vi "V1_controls.vi"() -> ()   [LabVIEW 2020]
uses:
  C:/Users/359167/Documents/LabVIEW_ws/Thorlabs.MotionControl.FTD2xx_Net.dll
  Thorlabs.MotionControl.FTD2xx_Net.dll
  <vilib>/DAQmx/read.llb/DAQmx Read (Analog 1D Wfm NChan NSamp).vi
panel:
  in  "Run":bool
  in  "End":bool
  out "Device ID":string[](array[string])
  out "Serial Number":string[](array[string])
  out "Voltage":dbl[][](array[numeric])
  out "Array":string[][](array[string])
  out "mount labels":string[](array[string])
  out "DAQ channels":string[](array[string])
  out "# of channels":i32
  out "voltage vs. time":waveform(dbl)[](graph) caption="data"
  out "# of mounts":i32
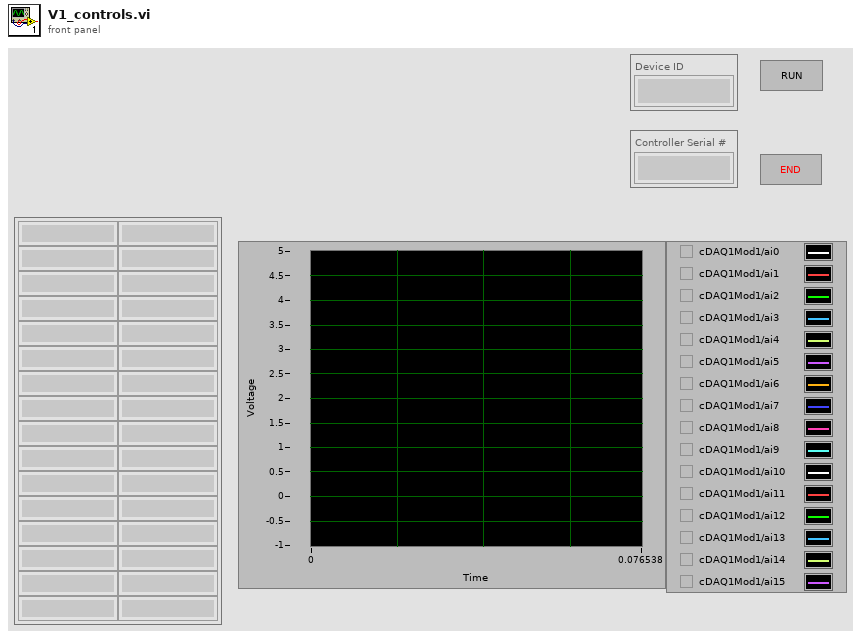
[diagram p1: front panel]
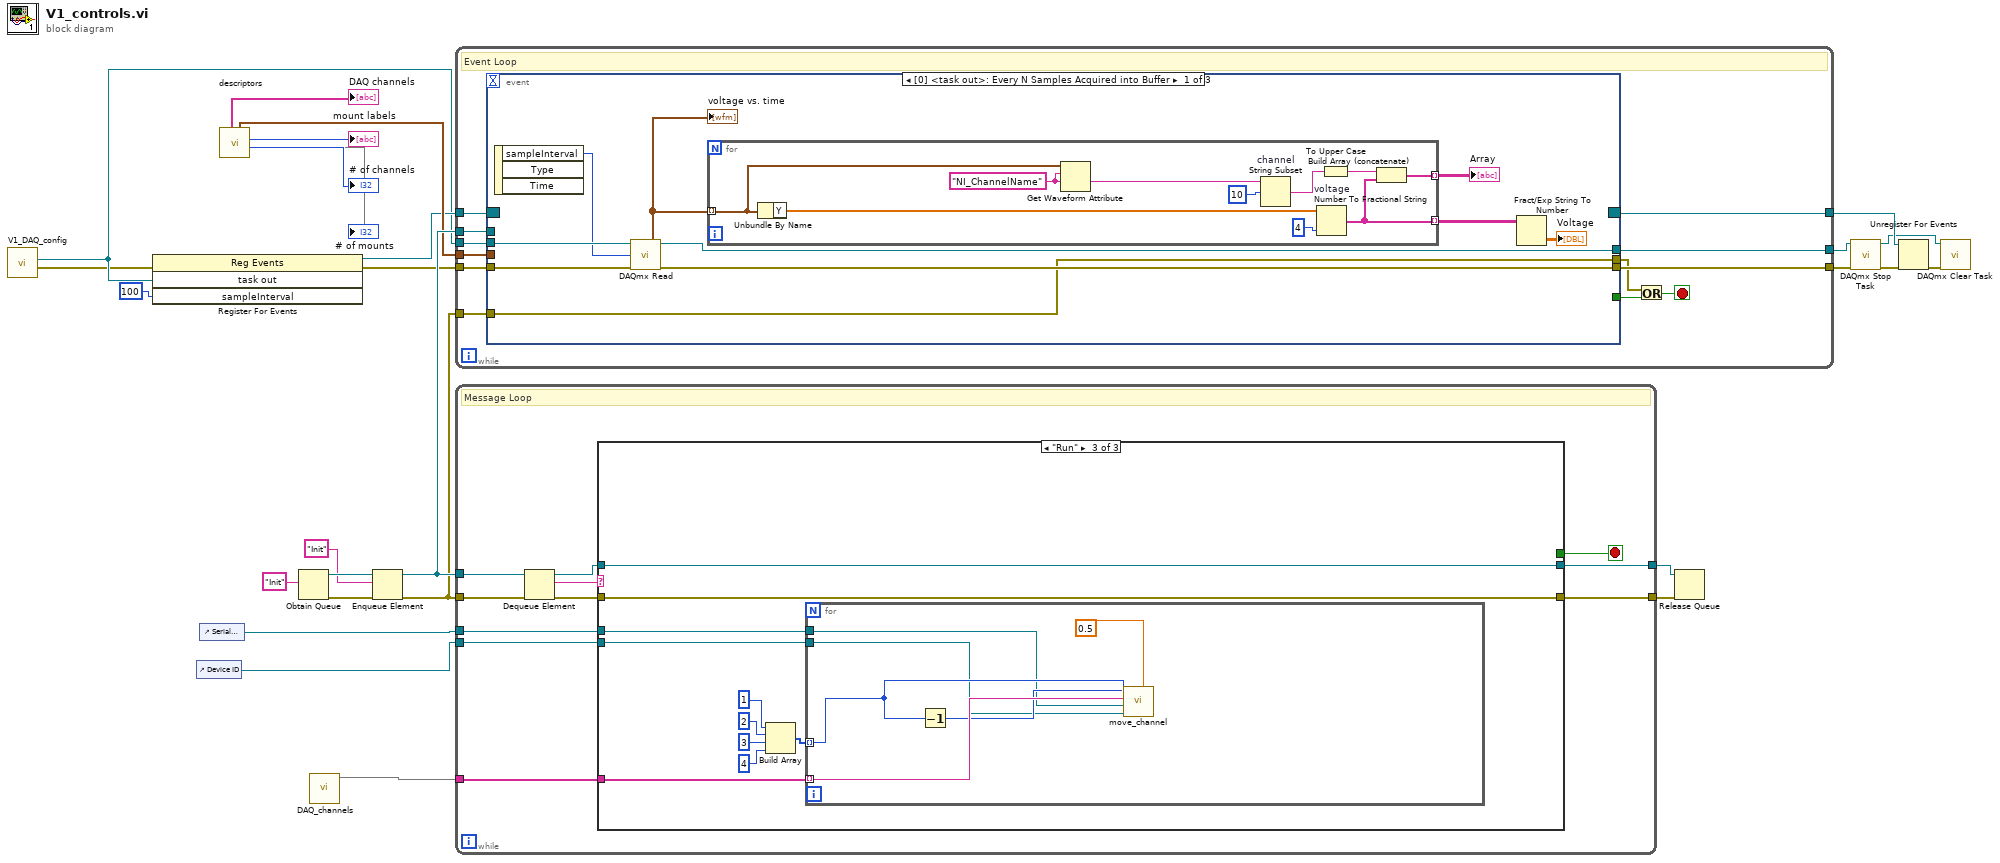
[diagram p0: block diagram]
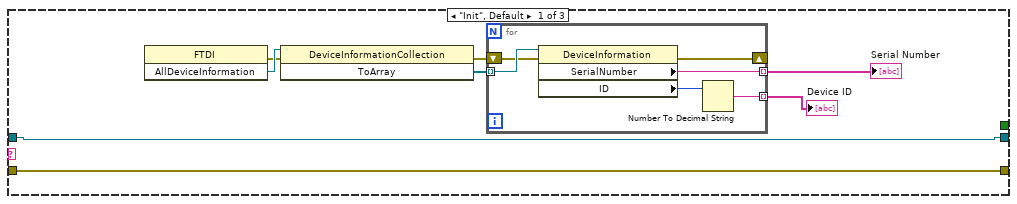
[diagram p2: hidden frame]
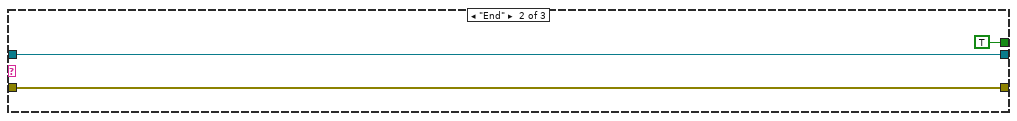
[diagram p3: hidden frame]
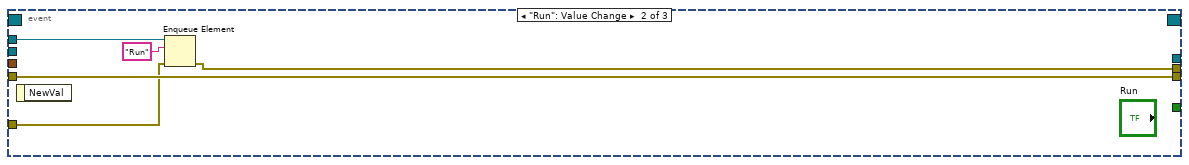
[diagram p4: hidden frame]
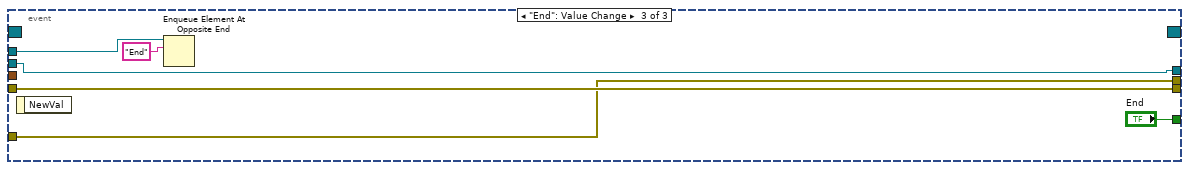
[diagram p5: hidden frame]
diagram:
  n1 = call "V1_DAQ_config.vi"() -> ("error out"=w7:errorcluster, "task out"=w12:refnum<k21>)  [unwired: 10 in]
  n2 = register-events(error in=w7, w12, u32 100 ("sampleInterval")) -> (reference out=w13:refnum<event-registration>, error out=w6:errorcluster)  [unwired: 1 in]
  n3 = control-ref of="Device ID"() -> (w1:refnum<vi>)
  n4 = control-ref of="Serial Number"() -> (w2:refnum<vi>)
  n5 = call "descriptors.vi"() -> ("# of channels"=→"# of channels":i32, "# of controllers"=→"mount labels":i32, 4:→"# of mounts", "channel pairs"=w21:cluster{i32, i32}[], "DAQ channels"=→"DAQ channels":string[])  [unwired: 6 in, 1 out]
  n6 = Obtain Queue(element data type="Init") -> (queue out=w26:refnum<queue>, error out=w27:errorcluster)  [unwired: 4 in, 1 out]
  n7 = call "DAQ_channels.vi"() -> (3:w4)  [unwired: 9 in, 2 out]
  n8 = Enqueue Element(queue=w26, element="Init", error in (no error)=w27) -> (queue out=w24:refnum<queue>, error out=w3:errorcluster)  [unwired: 1 in, 1 out]
  n9 = while {
    tunnel: w24 -> [w37]
    tunnel: w13 -> [w35]
    tunnel: w12 -> [w36]
    tunnel: [w34] -> w23
    tunnel: [w33] -> w22
    tunnel: w21 -> [w32]
    tunnel: w6 -> [w31]
    tunnel: [w30] -> w5
    tunnel: w3 -> [w29]
    stop <- w39 stop-if-true
    # "Event Loop"
    n10 = event shown="[0] <task out>: Every N Samples Acquired into Buffer" {
      selector: w35 -> [_ _ _]
      dyn-events: [_ _ _] -> w34
      timeout: _ -> [_ _ _]
      tunnel: [_ _ "End"] -> w38
      tunnel: w37 -> [_ w62 w70]
      tunnel: w36 -> [w49 _ w69]
      tunnel: [w48 _ w69] -> w33
      tunnel: w32 -> [_ _ _]
      tunnel: w31 -> [w42 w64 w66]
      tunnel: [w41 w64 w66] -> w30
      tunnel: w29 -> [w40 w61 w65]
      tunnel: [w40 w60 w65] -> w28
      event Every N Samples Acquired into Buffer {
        n11 = event-data() -> ("sampleInterval"=w47:u32)  [unwired: 1 in, 2 out]
        n12 = call-poly <vilib>:"DAQmx Read.vi"("task/channels in"=w49, "number of samples per channel"=w47, "error in"=w42) -> ("data"=w43:waveform(dbl)[], "task out"=w48:refnum<k21>, "error out"=w41:errorcluster)  [unwired: 10 in]
        "voltage vs. time" <- w43
        n13 = for {
          tunnel: w43 -> [w59] mode=indexing
          tunnel: [w53] -> w46 mode=indexing
          tunnel: [w50] -> w45 mode=indexing
          w58 = "NI_ChannelName" ("name")
          n14 = Unbundle By Name(w59) -> ("Y"=w51:dbl[])
          n15 = Get Waveform Attribute(5:w58, 6:w58, 7:w59) -> (1:w57:string)  [unwired: 1 in, 3 out]
          n16 = String Subset "channel"(string=w57, offset (0)=10) -> (substring=w55:string)  [unwired: 1 in]
          n17 = Number To Fractional String "voltage"(number=w51, precision (6)=i16 4) -> (F-format string=w50:string[])  [unwired: 2 in]
          n18 = To Upper Case(1:w55) -> (0:w54:string)
          n19 = Build Array (concatenate)(w54, w50) -> (w53:string[])
        }
        "Array" <- w46
        n20 = Fract/Exp String To Number(string=w45) -> (number=→"Voltage":dbl[][])  [unwired: 3 in, 1 out]
      }
      event "Run": Value Change {
        n21 = event-data() -> ()  [unwired: 1 in, 1 out]
        n22 = Enqueue Element(queue=w62, element="Run", error in (no error)=w61) -> (error out=w60:errorcluster)  [unwired: 1 in, 2 out]
      }
      event "End": Value Change {
        n23 = event-data() -> ()  [unwired: 1 in, 1 out]
        n24 = Enqueue Element At Opposite End(queue=w70, element="End") -> ()  [unwired: 2 in, 3 out]
      }
    }
    n25 = Or(x=w28, y=w38) -> (x .or. y?=w39:bool)
  }
  n26 = while {
    tunnel: w3 -> [w79]
    tunnel: w24 -> [w77]
    tunnel: [w75] -> w14
    tunnel: [w74] -> w15
    tunnel: w4 -> [w73]
    tunnel: w2 -> [w71]
    tunnel: w1 -> [w72]
    stop <- w81 stop-if-true
    # "Message Loop"
    n27 = Dequeue Element(queue=w77, error in (no error)=w79) -> (queue out=w78:refnum<queue>, element=w76:string, error out=w80:errorcluster)  [unwired: 1 in, 1 out]
    n28 = case shown="\"Run\"" w76 {
      tunnel: [_ TRUE _] -> w81
      tunnel: w80 -> [w84 w97 w107]
      tunnel: w78 -> [w82 w96 w108]
      tunnel: [w84 w97 w107] -> w75
      tunnel: [w82 w96 w108] -> w74
      tunnel: w73 -> [_ _ w101]
      tunnel: w72 -> [_ _ w100]
      tunnel: w71 -> [_ _ w99]
      frame "Init", Default {
        n29 = invoke class="FTDI" method="AllDeviceInformation"() -> (error out=w86:errorcluster, "AllDeviceInformation"=w88:refnum<k24>)  [unwired: 3 in, 1 out]
        n30 = invoke class="DeviceInformationCollection" method="ToArray"(reference=w88, error in=w86) -> (error out=w85:errorcluster, "ToArray"=w87:refnum<k24>[])  [unwired: 1 in, 1 out]
        n31 = for {
          tunnel: w87 -> [w95] mode=indexing
          shift-right: [w93] -> _
          shift-left: w85 -> [w94]
          tunnel: [w92] -> w89 mode=indexing
          tunnel: [w90] -> w83 mode=indexing
          n32 = property class="DeviceInformation"(reference=w95, error in=w94) -> (error out=w93:errorcluster, "SerialNumber"=w92:string, "ID"=w91:u32)  [unwired: 1 out]
          n33 = Number To Decimal String(number=w91) -> (decimal integer string=w90:string)  [unwired: 1 in]
        }
        "Serial Number" <- w89
        "Device ID" <- w83
      }
      frame "End" {
      }
      frame "Run" {
        n34 = Build Array(1, 2, 3, 4) -> (w102:i32[])
        n35 = for {
          tunnel: w102 -> [w112] mode=indexing
          tunnel: w101 -> [w114] mode=indexing
          tunnel: w100 -> [w110]
          tunnel: w99 -> [w109]
          n36 = Decrement(x=w112) -> (x-1=w111:i32)
          n37 = call "move_channel.vi"(5:0.5 ("Desired Position"), 7:w112, "Desired"=w110, "Device ID"=w109, "Serial #"=w114, "DAQ Channel"=w111) -> ()  [unwired: 3 in, 3 out]
        }
      }
    }
  }
  n38 = Release Queue(queue=w15, error in (no error)=w14) -> ()  [unwired: 1 in, 3 out]
  n39 = call <vilib>:"DAQmx Stop Task.vi"("task/channels in"=w22, "error in"=w5) -> ("task out"=w10:refnum<k21>, "error out"=w9:errorcluster)  [unwired: 12 in]
  n40 = Unregister For Events(event registration refnum=w23, error in=w9) -> (error out=w8:errorcluster)
  n41 = call <vilib>:"DAQmx Clear Task.vi"("task in"=w10, "error in"=w8) -> ()  [unwired: 13 in, 1 out]
